vi "Set Address.vi"(8 "error in (no error)":errorcluster, 10 "address":u64 format="%016x", 11 "Pointer in":refnum<class "Memory.Pointer.lvclass">) -> (0 "error out":errorcluster, 3 "Pointer out":refnum<class "Memory.Pointer.lvclass">)   [LabVIEW 2016, in "Memory Manager.lvlib" / "Memory.Pointer.lvclass"]
uses:
  Memory.Pointer.lvclass
  Memory.Pointer.lvclass/Memory.Pointer.ctl
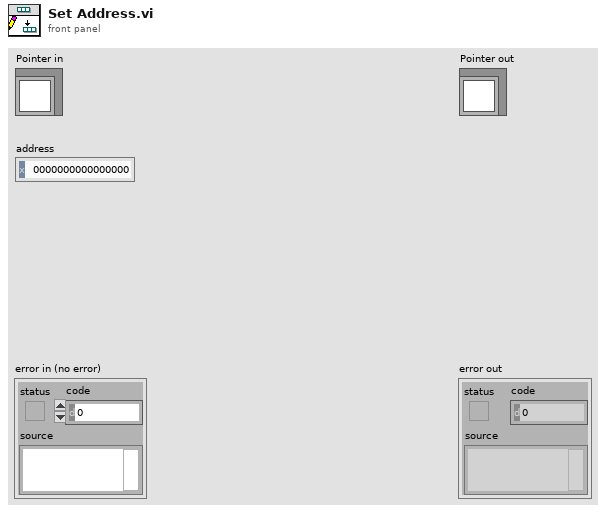
[diagram p1: front panel]
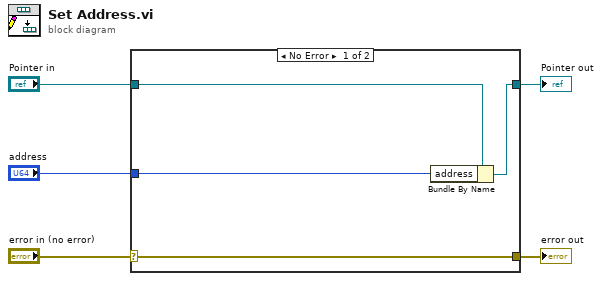
[diagram p0: block diagram]
diagram:
  n1 = case shown="No Error" "error in (no error)" {
    selector: "error in (no error)" -> [w9 w10]
    tunnel: [w9 w10] -> w4
    tunnel: [w7 w11] -> w2
    tunnel: "Pointer in" -> [w8 w11]
    tunnel: "address" -> [w6 _]
    frame No Error {
      n2 = Bundle By Name(cluster=w8, "address"=w6) -> (w7:refnum<class "Memory.Pointer.lvclass">)
    }
    frame Error {
    }
  }
  "error out" <- w4
  "Pointer out" <- w2
